vi "subVi solve.vi"(8 "error in (no error)":errorcluster, 11 "Rubix Array":T1[][](array[typedef])=[[{"Object Ref"=refnum, "Name"="r0"}, {"Object Ref"=refnum, "Name"="b0"}, {"Object Ref"=refnum, "Name"="o0"}, {"Object Ref"=refnum, "Name"="g0"}, {"Object Ref"=refnum, "Name"="y0"}, {"Object Ref"=refnum, "Name"="b1"}, {"Object Ref"=refnum, "Name"="g1"}, {"Object Ref"=refnum, "Name"="o1"}, {"Object Ref"=refnum, "Name"="y1"}], [{"Object Ref"=refnum, "Name"="w0"}, {"Object Ref"=refnum, "Name"="b2"}, {"Object Ref"=refnum, "Name"="g2"}, {"Object Ref"=refnum, "Name"="r1"}, {"Object Ref"=refnum, "Name"="o2"}, {"Object Ref"=refnum, "Name"="w1"}, {"Object Ref"=refnum, "Name"="b3"}, {"Object Ref"=refnum, "Name"="o3"}, {"Object Ref"=refnum, "Name"="o4"}], [{"Object Ref"=refnum, "Name"="r2"}, {"Object Ref"=refnum, "Name"="o5"}, {"Object Ref"=refnum, "Name"="r3"}, {"Object Ref"=refnum, "Name"="r4"}, {"Object Ref"=refnum, "Name"="w2"}, {"Object Ref"=refnum, "Name"="w3"}, {"Object Ref"=refnum, "Name"="g3"}, {"Object Ref"=refnum, "Name"="r5"}, {"Object Ref"=refnum, "Name"="g4"}], [{"Object Ref"=refnum, "Name"="y2"}, {"Object Ref"=refnum, "Name"="g5"}, {"Object Ref"=refnum, "Name"="w4"}, {"Object Ref"=refnum, "Name"="g6"}, {"Object Ref"=refnum, "Name"="r6"}, {"Object Ref"=refnum, "Name"="r7"}, {"Object Ref"=refnum, "Name"="o6"}, {"Object Ref"=refnum, "Name"="g7"}, {"Object Ref"=refnum, "Name"="y3"}], [{"Object Ref"=refnum, "Name"="b4"}, {"Object Ref"=refnum, "Name"="y4"}, {"Object Ref"=refnum, "Name"="w5"}, {"Object Ref"=refnum, "Name"="o7"}, {"Object Ref"=refnum, "Name"="b5"}, {"Object Ref"=refnum, "Name"="y5"}, {"Object Ref"=refnum, "Name"="b6"}, {"Object Ref"=refnum, "Name"="w6"}, {"Object Ref"=refnum, "Name"="b7"}], [{"Object Ref"=refnum, "Name"="r8"}, {"Object Ref"=refnum, "Name"="b8"}, {"Object Ref"=refnum, "Name"="o8"}, {"Object Ref"=refnum, "Name"="y6"}, {"Object Ref"=refnum, "Name"="g8"}, {"Object Ref"=refnum, "Name"="w7"}, {"Object Ref"=refnum, "Name"="w8"}, {"Object Ref"=refnum, "Name"="y7"}, {"Object Ref"=refnum, "Name"="y8"}]]) -> (0 "error out":errorcluster, 1 "Commands to Execute":string[](array[string]), 2 "Loesung":i32[](array[numeric]), 3 "Array":u16[][](array[numeric])=[[1, 5, 2, 4, 3, 5, 4, 2, 3], [0, 5, 4, 1, 2, 0, 5, 2, 2], [1, 2, 1, 1, 0, 0, 4, 1, 4], [3, 4, 0, 4, 1, 1, 2, 4, 3], [5, 3, 0, 2, 5, 3, 5, 0, 5], [1, 5, 2, 3, 4, 0, 0, 3, 3]])   [LabVIEW 2019]
uses:
  code solve/Rubix Array data type.ctl
  code solve/Rubik's Solver.dll
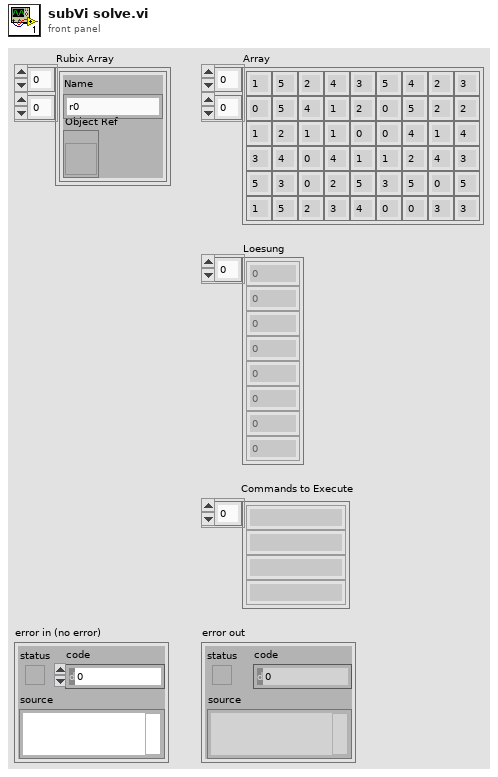
[diagram p1: front panel]
types:
  T1 = typedef "Rubix Array data type.ctl" = cluster{"Object Ref":refnum<vi>, "Name":string}
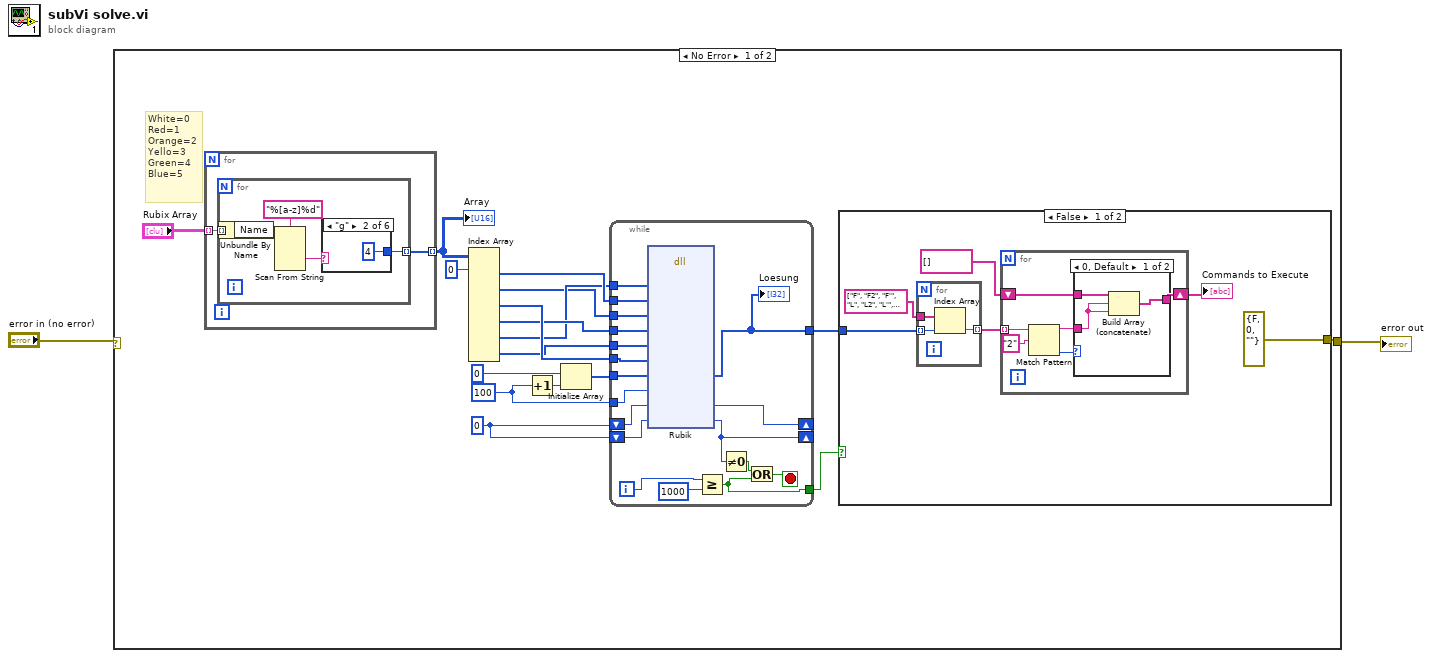
[diagram p0: block diagram]
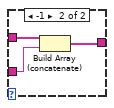
[diagram p2: hidden frame]
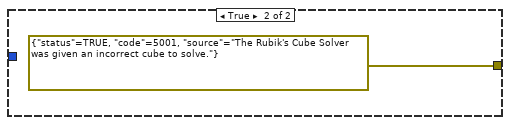
[diagram p3: hidden frame]
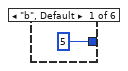
[diagram p4: hidden frame]
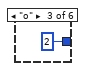
[diagram p5: hidden frame]
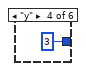
[diagram p6: hidden frame]
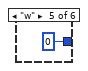
[diagram p7: hidden frame]
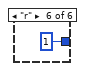
[diagram p8: hidden frame]
diagram:
  n1 = case shown="No Error" "error in (no error)" {
    selector: "error in (no error)" -> [_ w73]
    tunnel: [w3 w73] -> w2
    frame No Error {
      w15 = u8 0
      w16 = u16 100
      # "White=0\nRed=1\nOrange=2\nYello=3\nGreen=4\nBlue=5"
      n2 = for {
        tunnel: "Rubix Array" -> [w43] mode=indexing
        tunnel: [w42] -> w12 mode=indexing
        n3 = for {
          tunnel: w43 -> [w45] mode=indexing
          tunnel: [w46] -> w42 mode=indexing
          n4 = Unbundle By Name(w45) -> ("Name"=w44:string)
          n5 = Scan From String(format string="%[a-z]%d", input string=w44) -> (output 1=w48:string)  [unwired: 5 in, 3 out]
          n6 = case shown="\"g\"" w48 {
            tunnel: [u16 5 u16 4 u16 2 u16 3 u16 0 u16 1] -> w46
            frame "b", Default {
            }
            frame "g" {
            }
            frame "o" {
            }
            frame "y" {
            }
            frame "w" {
            }
            frame "r" {
            }
          }
        }
      }
      "Array" <- w12
      n7 = Index Array(array=w12, index (row) #1=0 ("disabled index (col)")) -> (element #1=w10:u16[], element #2=w5:u16[], element #3=w9:u16[], element #4=w8:u16[], element #5=w7:u16[], element #6=w6:u16[])  [unwired: 11 in]
      n8 = Increment(x=w16) -> (x+1=w18:u16)
      n9 = Initialize Array(0 ("element"), w18) -> (w17:i32[])
      n10 = while {
        tunnel: w17 -> [w72]
        shift-right: [w68] -> _
        shift-left: w15 -> [w71]
        tunnel: w16 -> [w67]
        shift-right: [w69] -> _
        shift-left: w15 -> [w70]
        tunnel: [w60] -> w11
        tunnel: w7 -> [w66]
        tunnel: w10 -> [w65]
        tunnel: w5 -> [w64]
        tunnel: w8 -> [w63]
        tunnel: w6 -> [w62]
        tunnel: w9 -> [w61]
        tunnel: [w55] -> w4
        i -> [w59]
        stop <- w56 stop-if-true
        n11 = dll-call lib="D:/rubix/code solve/Rubik's Solver.dll" fn="Rubik"("Up"=w66, "Front"=w65, "Right"=w64, "Left"=w63, "Down"=w62, "Back"=w61, "Loesung"=w72, "Anzahl"=w67, "Error"=w70, "ready"=w71) -> ("Loesung"=w60:i32[], "Error"=w69:u8, "ready"=w68:u8)  [unwired: 11 in, 2 out]
        "Loesung" <- w60
        n12 = Greater Or Equal?(x=w59, y=1000 ("x")) -> (x >= y?=w55:bool)
        n13 = Not Equal To 0?(x=w68) -> (x != 0?=w57:bool)
        n14 = Or(x=w57, y=w55) -> (x .or. y?=w56:bool)
      }
      n15 = case shown="False" w4 {
        tunnel: w11 -> [w23 _]
        tunnel: [errorcluster {"status"=FALSE, "code"=0, "source"=""} ("error IO") errorcluster {"status"=TRUE, "code"=5001, "source"="The Rubik's Cube Solver  was given an incorrect cube to solve."} ("error IO")] -> w3
        frame False {
          n16 = for {
            tunnel: w23 -> [w40] mode=indexing
            tunnel: [w39] -> w25 mode=indexing
            tunnel: string[] ["F", "F2", "F'", "L", "L2", "L'", "U", "U2", "U'", "B", "B2", "B'", "R", "R2", "R'", "D", "D2", "D'"] -> [w38]
            n17 = Index Array(array=w38, index=w40) -> (element=w39:string)
          }
          n18 = for {
            tunnel: w25 -> [w31] mode=indexing
            shift-right: [w26] -> w21
            shift-left: string[] [] -> [w27]
            n19 = Match Pattern(string=w31, regular expression="2") -> (before substring=w28:string, offset past match=w29:i32)  [unwired: 1 in, 2 out]
            n20 = case shown="0, Default" w29 {
              tunnel: w28 -> [w32 w35]
              tunnel: w27 -> [w34 w37]
              tunnel: [w33 w36] -> w26
              frame 0, Default {
                n21 = Build Array (concatenate)(w34, w32, w32) -> (w33:string[])
              }
              frame -1 {
                n22 = Build Array (concatenate)(w37, w35) -> (w36:string[])
              }
            }
          }
          "Commands to Execute" <- w21
        }
        frame True {
        }
      }
    }
    frame Error {
    }
  }
  "error out" <- w2
